vi "Line Detector Crop Regions.vi"(6 "Region width":dbl=500000.0 format="%#_6pHz", 7 "Frequency":dbl[](array[numeric]), 9 "Magnitude":dbl[](array[numeric]), 10 "Signal":cdb[](array[numeric]), 11 "Best fit":dbl[][](array[numeric]) format="%#_4p") -> (2 "Regions signals":waveform(cdb)[](array[waveform]), 3 "Regions frequencies":waveform(dbl)[](array[waveform]))   [LabVIEW 2020]
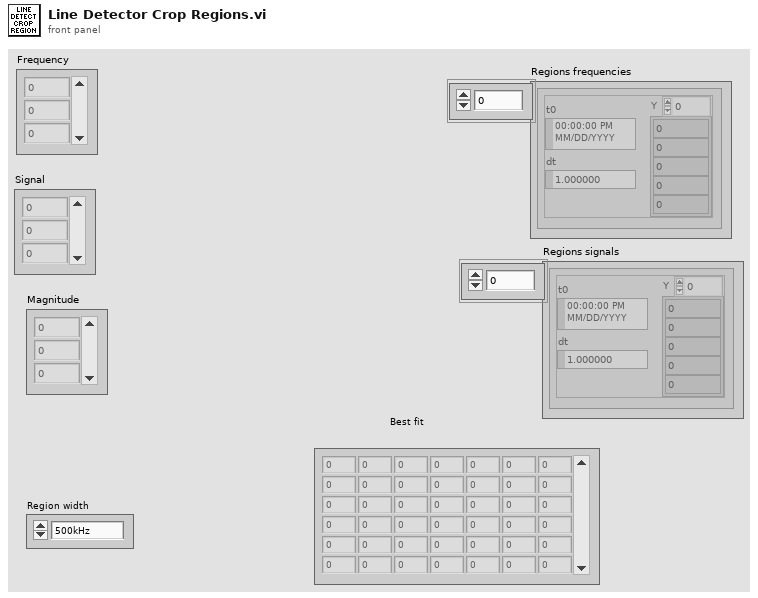
[diagram p1: front panel]
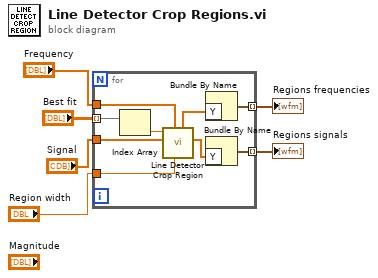
[diagram p0: block diagram]
diagram:
  n1 = for {
    tunnel: "Best fit" -> [w15] mode=indexing
    tunnel: "Frequency" -> [w11]
    tunnel: "Signal" -> [w13]
    tunnel: "Region width" -> [w12]
    tunnel: [w9] -> w1 mode=indexing
    tunnel: [w8] -> w2 mode=indexing
    n2 = Index Array(array=w15) -> (element=w14:dbl)  [unwired: 1 in]
    n3 = call "Line Detector Crop Region.vi"("Region width"=w12, "Frequency"=w11, "Signal"=w13, "Center frequency"=w14) -> ("Signal  out"=w10:cdb[], "Frequency out"=w7:dbl[])  [unwired: 4 in, 2 out]
    n4 = Bundle By Name("Y"=w7) -> (w8:waveform(dbl))  [unwired: 1 in]
    n5 = Bundle By Name("Y"=w10) -> (w9:waveform(cdb))  [unwired: 1 in]
  }
  "Regions signals" <- w1
  "Regions frequencies" <- w2
